vi "Request Message.vi"(6 "timeout in ms (-1)":i32=-1, 8 "error in (no error)":errorcluster, 9 "Request Message Data":variant, 10 "Request Message":string, 11 "Process In":refnum<class "Debug Process.lvclass">) -> (0 "error out":errorcluster, 1 "Response Message Data":variant, 2 "Response Message":string, 3 "Process Out":refnum<class "Debug Process.lvclass">, 4 "Timed out?":bool)   [LabVIEW 2020, in "Debug Process.lvclass"]
doc: "Make a syncronous request to the process. The process must respond to the request made using the Response Message.vi method within the configured timeout period to avoid this method from timing out. \nThis method will throw an error if called within the own process loop.\n\nTo implement an asynchronous request, call the request within the Asynchronous Action interface and message the process when the request has returned."
uses:
  Debug Process.lvclass
  Debug Process.lvclass/Debug Process.ctl
  <vilib>/Utility/error.llb/Clear Errors.vi
  <vilib>/Utility/error.llb/Error Cluster From Error Code.vi
  <vilib>/ErrorRing/Error Ring.xnode
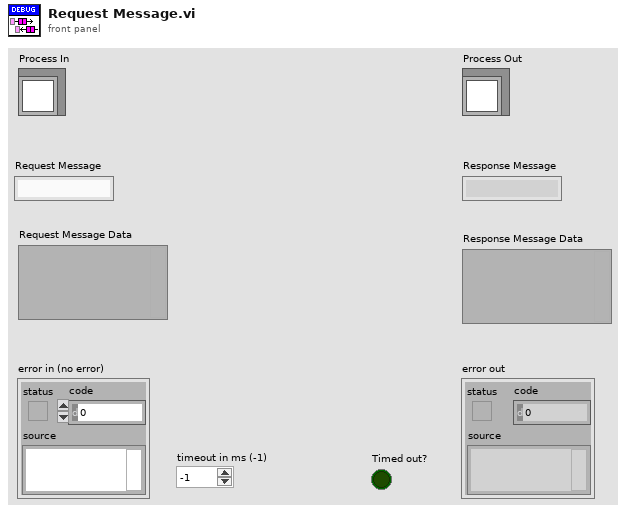
[diagram p1: front panel]
types:
  T1 = typedef "Debug Process.lvclass/Lifecycle State.ctl" = enum16{"Uninitialized", "Initialized", "Started", "Running", "Stopped", "Finished"}
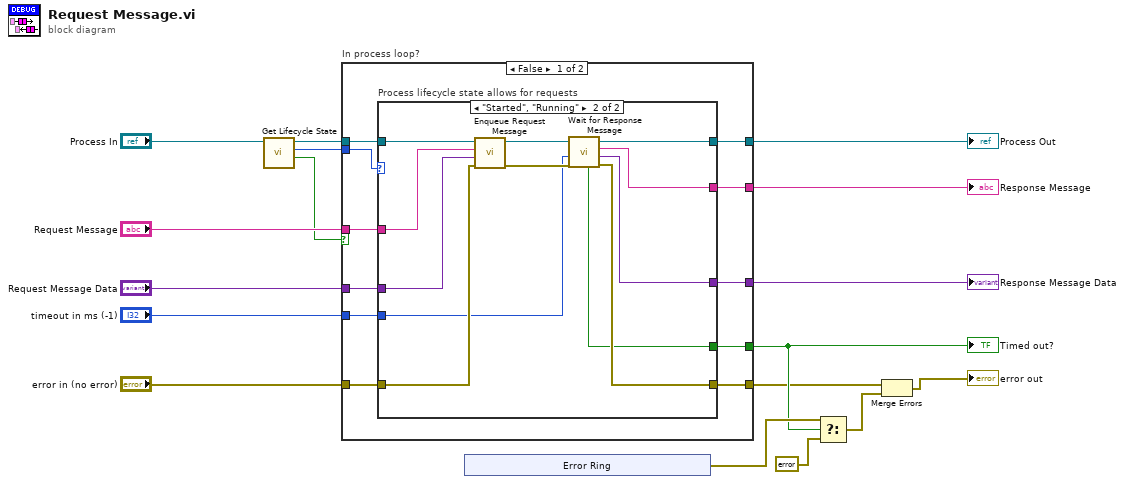
[diagram p0: block diagram]
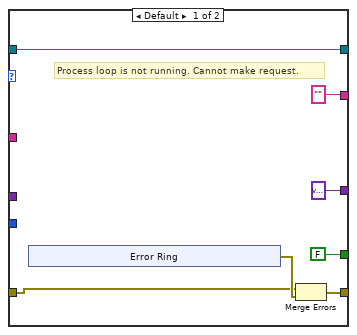
[diagram p2: hidden frame]
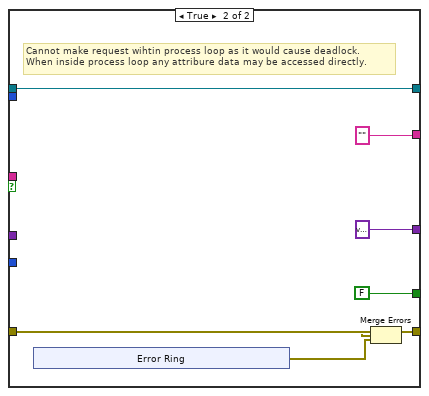
[diagram p3: hidden frame]
diagram:
  n1 = call "Get Lifecycle State.vi"("Process In"="Process In") -> ("In Process Loop?"=w3:bool, "Lifecycle State"=w2:T1, "Process Out"=w4:refnum<class "Debug Process.lvclass">)  [unwired: 7 in, 1 out]
  n2 = case "In process loop?" shown="False" w3 {
    tunnel: "Request Message" -> [w28 _]
    tunnel: "Request Message Data" -> [w27 _]
    tunnel: [w26 w58] -> w15
    tunnel: "timeout in ms (-1)" -> [w25 _]
    tunnel: [w24 w53] -> w10
    tunnel: w4 -> [w23 w58]
    tunnel: "error in (no error)" -> [w22 w54]
    tunnel: [w21 FALSE ("timed out?")] -> w11
    tunnel: [w20 "" ("Message")] -> w8
    tunnel: [w19 variant ("Message Data")] -> w9
    tunnel: w2 -> [w18 _]
    frame False {
      n3 = case "Process lifecycle state allows for requests" shown="\"Started\", \"Running\"" w18 {
        tunnel: w28 -> [_ w51]
        tunnel: w27 -> [_ w50]
        tunnel: [w29 w42] -> w26
        tunnel: w25 -> [_ w41]
        tunnel: [w33 w47] -> w24
        tunnel: w23 -> [w29 w45]
        tunnel: w22 -> [w34 w44]
        tunnel: [FALSE ("timed out?") w40] -> w21
        tunnel: ["" ("Message") w49] -> w20
        tunnel: [variant ("Message Data") w48] -> w19
        frame Default {
          # "Process loop is not running. Cannot make request."
          n4 = xnode "Error Ring"() -> ("error out"=w35:errorcluster)
          n5 = Merge Errors(w34, w35) -> (w33:errorcluster)
        }
        frame "Started", "Running" {
          n6 = call "Enqueue Request Message.vi"("error in (no error)"=w44, "Message Data"=w50, "Message"=w51, "Process In"=w45) -> ("error out"=w43:errorcluster, "Process Out"=w46:refnum<class "Debug Process.lvclass">)  [unwired: 6 in]
          n7 = call "Wait for Response Message.vi"("error in (no error)"=w43, "timeout in ms"=w41, "Process In"=w46) -> ("error out"=w47:errorcluster, "Message Data"=w48:variant, "Message"=w49:string, "Process Out"=w42:refnum<class "Debug Process.lvclass">, "timed out?"=w40:bool)  [unwired: 4 in]
        }
      }
    }
    frame True {
      # "Cannot make request wihtin process loop as it would cause deadlock.\nWhen inside process loop any attribure data may be accessed directly."
      n8 = xnode "Error Ring"() -> ("error out"=w52:errorcluster)
      n9 = Merge Errors(w54, w52) -> (w53:errorcluster)
    }
  }
  "Process Out" <- w15
  "Response Message" <- w8
  "Response Message Data" <- w9
  "Timed out?" <- w11
  n10 = xnode "Error Ring"() -> ("error out"=w12:errorcluster)
  n11 = Select(t=w12, s=w11, f=errorcluster {"status"=FALSE, "code"=0, "source"=""}) -> (s? t:f=w7:errorcluster)
  n12 = Merge Errors(w10, w7) -> (→"error out":errorcluster)
